vi "Stop Measurements.vi"(6 "Controller name":string, 8 "error in (no error)":errorcluster, 10 "Request type":T1, 11 "Measure Controller in":refnum<class "Process Controller.lvclass">) -> (0 "error out":errorcluster, 3 "Measure Controller out":refnum<class "Process Controller.lvclass">)   [LabVIEW 2021, in "Process Controller.lvclass"]
uses:
  Process Controller.lvclass
  C:/GitHub/LabActor/Worker/Worker.lvclass
  C:/Program Files/National Instruments/LabVIEW 2021/vi.lib/ActorFramework/Actor/Actor.lvclass
  Request type.ctl
  Worker/Worker.lvclass/Worker.ctl
  NHMFL_Core/Libraries/Instruments/Instrument Driver/Worker State.ctl
  Process Controller Messages/Stop Response Msg/Stop Response Msg.lvclass
  C:/GitHub/LabActor/Template Module Messages/Self-Addressed Msg/Self-addressed Msg.lvclass
  Process Controller.lvclass/Process Controller.ctl
  <vilib>/ActorFramework/Actor/Actor.lvclass/Actor.ctl
  <vilib>/ActorFramework/Message Enqueuer/Message Enqueuer.lvclass/Message Enqueuer.ctl
  Template Module Messages/Self-Addressed Msg/Self-addressed Msg.lvclass/Self-addressed Msg.ctl
  Worker Messages/Stop Work Msg/Stop Work Msg.lvclass/Stop Work Msg.ctl
  Template Module/Write State.vi
  Read Active measurements enqueuers.vi
  Worker/Write Pause requested.vi
  Worker/Write Paused.vi
  Template Module Messages/Self-Addressed Msg/Write Return Enqueuer.vi
  Template Module/Read State.vi
  <vilib>/ActorFramework/Message Enqueuer/Init from Existing Queue.vi
  <vilib>/ActorFramework/Message Enqueuer/Enqueue.vi
  Worker Messages/Stop Work Msg/Stop Work Msg.lvclass
  C:/Program Files/National Instruments/LabVIEW 2021/vi.lib/ActorFramework/Message/Message.lvclass
  <vilib>/ActorFramework/Message Priority Queue/Priority Enqueue.vi
  <vilib>/ActorFramework/Message Enqueuer/Message Enqueuer.lvclass
  <vilib>/ActorFramework/Actor/Actor.lvclass
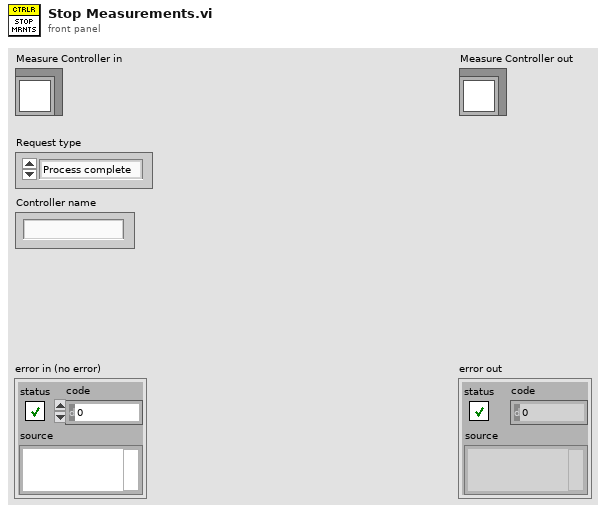
[diagram p1: front panel]
types:
  T1 = typedef "Request type.ctl" = enum16{"Process complete", "User command", "Auto-restart", "Error"}
  T2 = typedef "Worker State.ctl" = enum16{"Idle", "Starting", "Working", "Stopping"}
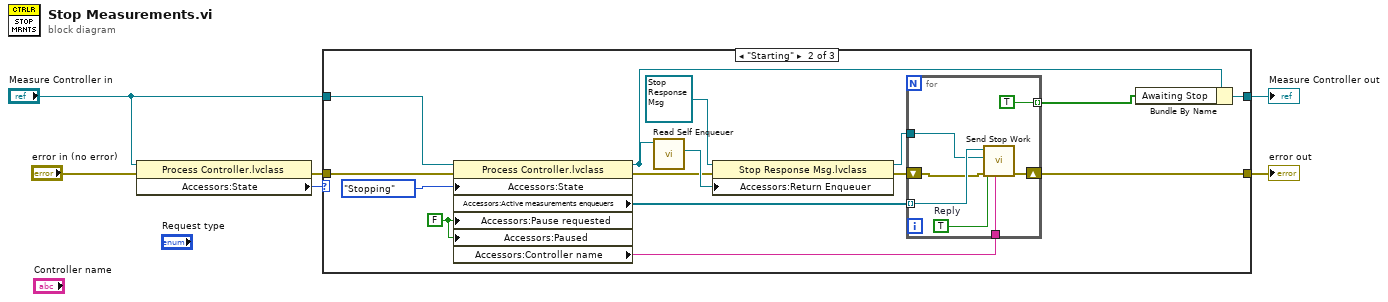
[diagram p0: block diagram]
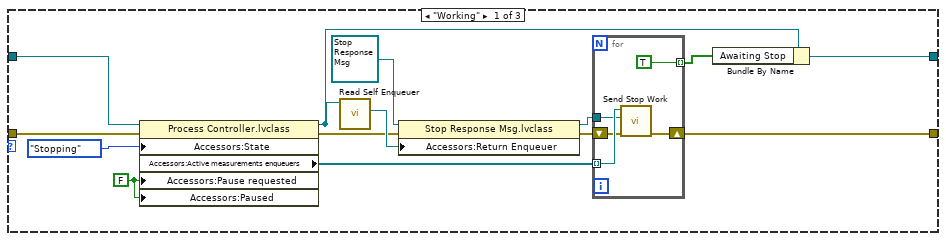
[diagram p2: hidden frame]
diagram:
  n1 = property class="Process Controller.lvclass"(reference="Measure Controller in", error in="error in (no error)") -> (error out=w1:errorcluster, "Accessors:State"=w2:T2)  [unwired: 1 out]
  n2 = case shown="\"Starting\"" w2 {
    tunnel: [w19 w39 w48] -> w6
    tunnel: [w9 w29 w49] -> w5
    tunnel: "Measure Controller in" -> [w20 w40 w49]
    tunnel: w1 -> [w10 w30 w48]
    frame "Working" {
      w7 = FALSE ("Pause requested")
      n3 = property class="Process Controller.lvclass"(reference=w20, error in=w10, "Accessors:State"=Worker_State."Stopping" ("State"), "Accessors:Pause requested"=w7, "Accessors:Paused"=w7) -> (reference out=w16:refnum<class "Process Controller.lvclass">, error out=w13:errorcluster, "Accessors:Active measurements enqueuers"=w18:refnum<class "Message Enqueuer.lvclass">[])
      n4 = call <vilib>:"Read Self Enqueuer.vi"("Actor"=w16) -> ("Self Enqueuer"=w14:refnum<class "Message Enqueuer.lvclass">)  [unwired: 10 in]
      n5 = property class="Stop Response Msg.lvclass"(reference=refnum<class "Stop Response Msg.lvclass"> refnum ("Stop Response Msg.lvclass"), error in=w13, "Accessors:Return Enqueuer"=w14) -> (reference out=w12:refnum<class "Stop Response Msg.lvclass">, error out=w11:errorcluster)
      n6 = for {
        tunnel: w18 -> [w25] mode=indexing
        shift-right: [w23] -> w19
        shift-left: w11 -> [w24]
        tunnel: w12 -> [w22]
        tunnel: [TRUE] -> w8 mode=indexing
        n7 = call "Send Stop Work.vi"("error in (no error)"=w24, "Reply to"=w22, "Message Enqueuer"=w25) -> ("error out"=w23:errorcluster)  [unwired: 7 in, 1 out]
      }
      n8 = Bundle By Name(cluster=w16, "Awaiting Stop"=w8) -> (w9:refnum<class "Process Controller.lvclass">)
    }
    frame "Starting" {
      w27 = FALSE ("Pause requested")
      n9 = property class="Process Controller.lvclass"(reference=w40, error in=w30, "Accessors:State"=Worker_State."Stopping" ("State"), "Accessors:Pause requested"=w27, "Accessors:Paused"=w27) -> (reference out=w36:refnum<class "Process Controller.lvclass">, error out=w33:errorcluster, "Accessors:Active measurements enqueuers"=w38:refnum<class "Message Enqueuer.lvclass">[], "Accessors:Controller name"=w26:string)
      n10 = call <vilib>:"Read Self Enqueuer.vi"("Actor"=w36) -> ("Self Enqueuer"=w34:refnum<class "Message Enqueuer.lvclass">)  [unwired: 10 in]
      n11 = property class="Stop Response Msg.lvclass"(reference=refnum<class "Stop Response Msg.lvclass"> refnum ("Stop Response Msg.lvclass"), error in=w33, "Accessors:Return Enqueuer"=w34) -> (reference out=w32:refnum<class "Stop Response Msg.lvclass">, error out=w31:errorcluster)
      n12 = for {
        tunnel: w38 -> [w47] mode=indexing
        shift-right: [w45] -> w39
        shift-left: w31 -> [w46]
        tunnel: w32 -> [w44]
        tunnel: [TRUE] -> w28 mode=indexing
        tunnel: w26 -> [w41]
        w42 = TRUE  # Reply
        n13 = call "Send Stop Work.vi"("Controller name"=w41, "error in (no error)"=w46, "Reply"=w42, "Reply to"=w44, "Message Enqueuer"=w47) -> ("error out"=w45:errorcluster)  [unwired: 5 in, 1 out]
      }
      n14 = Bundle By Name(cluster=w36, "Awaiting Stop"=w28) -> (w29:refnum<class "Process Controller.lvclass">)
    }
    frame "Idle", Default {
    }
  }
  "error out" <- w6
  "Measure Controller out" <- w5
